vi "Prepare For Read Many.vi"(8 "error in (no error)":errorcluster, 10 "Minimum Call Pool Size":i32) -> (0 "error out":errorcluster, 3 "VI out":refnum<vi>)   [LabVIEW 2017, in "Futures.lvlib" / "Future.lvclass"]
uses:
  Future.lvclass
  Indexed Read.vi
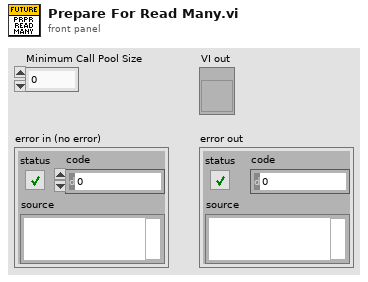
[diagram p1: front panel]
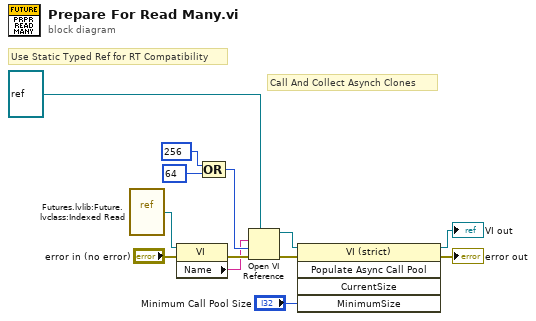
[diagram p0: block diagram]
diagram:
  # "Call And Collect Asynch Clones"
  # "Use Static Typed Ref for RT Compatibility"
  n1 = vi-ref "Futures.lvlib:Future.lvclass:Indexed Read.vi"() -> (w1:refnum<vi>)
  n2 = property class="VI"(reference=w1, error in="error in (no error)") -> (error out=w8:errorcluster, "Name"=w2:string)  [unwired: 1 out]
  n3 = Compound Arithmetic op=OR(256 ("options"), 64 ("options")) -> (w4:i32)
  n4 = Open VI Reference(type specifier VI Refnum (for type only)=refnum<vi> refnum, vi path=w2, options=w4, error in (no error)=w8) -> (vi reference=w9:refnum<vi>, error out=w10:errorcluster)  [unwired: 2 in]
  n5 = invoke class="VI (strict)" method="Populate Async Call Pool"(reference=w9, error in=w10, "MinimumSize"="Minimum Call Pool Size") -> (reference out=→"VI out":refnum<vi>, error out=→"error out":errorcluster)  [unwired: 2 in, 3 out]
